vi "Stop Core.vi"(10 "final error code":i32, 11 "VolatusCore in":refnum<class "VolatusCore.lvclass">) -> (3 "VolatusCore out":refnum<class "VolatusCore.lvclass">)   [LabVIEW 2020, in "Volatus.lvlib" / "VolatusCore.lvclass"]
doc: "(<B>Filename</B>: Actor Framework.lvlib:Actor.lvclass:Stop Core.vi)\n\nDefines what the actor does before it stops. Use the <B>final error code</B> input to determine whether the actor shut down in response to an error.\n\nBy default, this method passes the Stop message along to all auto-stop nested actors. A descendant class may override this method to define additional behavior, such as shutting down any processes the actor initiated in its override of the Actor Core method."
uses:
  VolatusCore.lvclass
  VolatusCore.lvclass/VolatusCore.ctl
  <vilib>/ActorFramework/Actor/Actor.lvclass
  App/App.lvclass
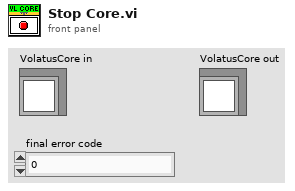
[diagram p1: front panel]
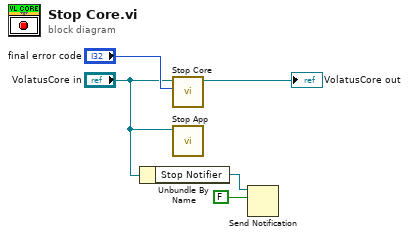
[diagram p0: block diagram]
diagram:
  n1 = Unbundle By Name("VolatusCore in") -> ("Stop Notifier"=w2:refnum<notifier>)
  n2 = call-parent "Stop Core.vi"("final error code"="final error code", "Actor in"="VolatusCore in") -> ("Actor out"=→"VolatusCore out":refnum<class "VolatusCore.lvclass">)  [unwired: 9 in]
  n3 = call "Stop App.vi"("VolatusCore in"="VolatusCore in") -> ()  [unwired: 9 in, 2 out]
  n4 = Send Notification(notification=FALSE, notifier=w2) -> ()  [unwired: 1 in, 2 out]
